vi "Do.vi"(8 "error in (no error)":errorcluster, 10 "Actor in":refnum<class "Actor.lvclass">, 11 "Clear Arbitrary Sequence [SEQ] Msg":refnum<class "Clear Arbitrary Sequence [SEQ] Msg.lvclass">) -> (0 "error out":errorcluster, 2 "Actor out":refnum<class "Actor.lvclass">)   [LabVIEW 2014, in "CS++Fgen.lvlib" / "Clear Arbitrary Sequence [SEQ] Msg.lvclass"]
doc: "This VI delivers the message to the actor by calling the appropriate method(s) on the actor."
uses:
  Clear Arbitrary Sequence [SEQ] Msg.lvclass
  <vilib>/ActorFramework/Actor/Actor.lvclass
  CS++Fgen/CS++Fgen.lvclass
  CSPP_Core/Actors/CS++PVMonitor Messages/CS++PVUpdate Msg/CS++PVUpdate Msg.lvclass/CS++PVUpdate Msg.ctl
  CSPP_Core/Classes/CS++ProcessVariables/ProcessVariable/PV.lvclass/PV.ctl
  Clear Arbitrary Sequence [SEQ] Msg.lvclass/Clear Arbitrary Sequence [SEQ] Msg.ctl
  CSPP_Core/Classes/CS++ProcessVariables/ProcessVariable/PV.lvclass
  CSPP_Core/Actors/CS++PVMonitor Messages/CS++PVUpdate Msg/CS++PVUpdate Msg.lvclass
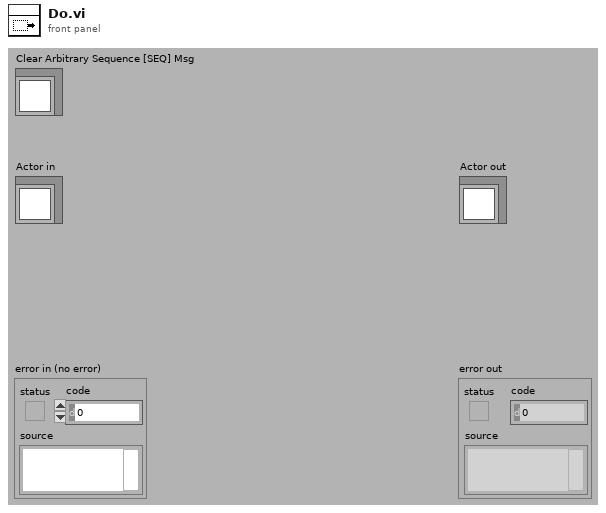
[diagram p1: front panel]
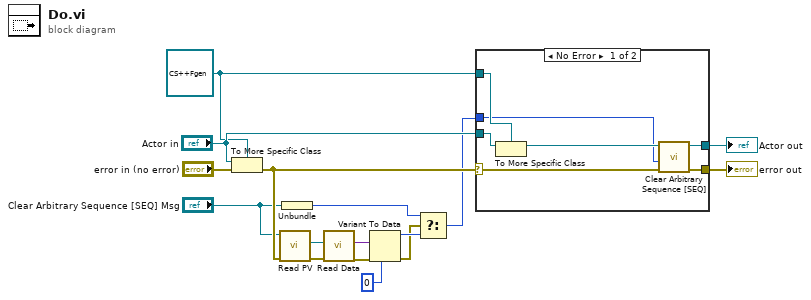
[diagram p0: block diagram]
diagram:
  w12 = refnum<class "CS++Fgen.lvclass"> refnum ("Actor in")
  n1 = To More Specific Class(target class=w12, reference="Actor in", error in="error in (no error)") -> (error out=w5:errorcluster)  [unwired: 1 out]
  n2 = call "Read PV.vi"("error in (no error)"=w5, "CS++PVUpdate Msg in"="Clear Arbitrary Sequence [SEQ] Msg") -> ("error out"=w8:errorcluster, "PV"=w11:refnum<class "PV.lvclass">)  [unwired: 7 in, 1 out]
  n3 = Unbundle("Clear Arbitrary Sequence [SEQ] Msg") -> (w2:i32)
  n4 = call "Read Data.vi"("error in (no error)"=w8, "PV in"=w11) -> ("error out"=w7:errorcluster, "Data"=w9:variant)  [unwired: 7 in, 1 out]
  n5 = Variant To Data(error in=w7, type=0, Variant=w9) -> (data=w10:i32, error out=w6:errorcluster)
  n6 = Select(t=w2, s=w6, f=w10) -> (s? t:f=w1:i32)
  n7 = case shown="No Error" w5 {
    selector: w5 -> [w21 w25]
    tunnel: [w23 w25] -> w15
    tunnel: [w22 w24] -> w14
    tunnel: "Actor in" -> [w20 w24]
    tunnel: w12 -> [w19 _]
    tunnel: w1 -> [w17 _]
    frame No Error {
      n8 = To More Specific Class(target class=w19, reference=w20) -> (specific class reference=w18:refnum<class "CS++Fgen.lvclass">)  [unwired: 1 in, 1 out]
      n9 = call "Clear Arbitrary Sequence [SEQ].vi"("error in (no error)"=w21, "sequence handle (0)"=w17, "CS++Fgen in"=w18) -> ("error out"=w23:errorcluster, "CS++Fgen out"=w22:refnum<class "CS++Fgen.lvclass">)  [unwired: 7 in]
    }
    frame Error {
      # "If type check fails, pass the original object out again."
    }
  }
  "error out" <- w15
  "Actor out" <- w14
